vi "Fetch Multiple Records.vi"(0 "device session in":refnum<class "Device Session.lvclass">, 1 "starting record":u64, 2 "number of records":u64=1, 5 "fetch relative to":T1=enum."First Pretrigger Sample", 7 "number of samples":u64=1000, 9 "timeout (ms)":i32=1000, 11 "error in":errorcluster, 12 "fetch offset":i64) -> (4 "device session out":refnum<class "Device Session.lvclass">, 6 "data":dbl[][](array[numeric]), 8 "relativeX (samples)":dbl[](array[numeric]), 14 "requested records info":T2[](array[typedef]), 15 "error out":errorcluster)   [LabVIEW 2021, in "Device Session.lvclass"]
doc: "Fetches data from multiple records in an acquisition. No data is returned if this VI times out. You must run the <B>Initiate</B> VI before running this VI.\n\n<B>Input Parameters</B>\n\n<B>device session in</B> is a reference to the Device Session object, which contains a session to each instrument design library used in this sample project. This parameter is obtained from the 'Open Session' VI.\n\n<B>number of records</B> specifies the number of records to fetch samples from. The default value is 1.\n\n<B>starting record</B> specifies the record to retrieve. Index of the record numbers starts at 0.\n\n<B>fetch relative to</B> specifies the relative location within the acquired record from where the VI begins to fetch data.\n\n'First Sample': the fetch starts at the first sample acquired by the device. If the device wraps data in its memory buffer, the first sample is no longer available. In this case, the VI returns an error if 'fetch offset' specifies a location that is within the overwritten portion of the memory buffer.\n'Reference Trigger Sample': the fetch starts relative to the Reference Trigger.\n'First Pretrigger Sample': the fetch starts relative to the first pretrigger sample acquired. If you do not configure a Reference Trigger, 'First Pretrigger Sample' behaves the same as 'First Sample' because there are no pretrigger samples.\n'Most Recent Sample': the fetch starts relative to the most recently acquired sample. The value of 'fetch offset' must be negative. This VI doesn't support this option. Consider using the 'Fetch Single Record' VI instead.\n'Current Read Position': the fetch starts after the last fetched sample. This VI doesn't support this option. Consider using the 'Fetch Single Record' VI instead.\n\n<B>number of samples</B> specifies the number of samples to fetch. The default value is 1000.\n\n<B>timeout (ms)</B> specifies the time, in milliseconds, allotted for the Fetch Multiple Records VI to complete execution of each record before returning a timeout error. A value of -1 specifies that the VI waits until all data is available. A value of 0 is not supported. The default value is 10,000. You cannot abort a pending fetch using the Abort VI or Close VI.\n\n<B>fetch offset</B> specifies the offset relative to the position, which is specified by the 'fetch relative to' parameter, from which to start fetching data. Offset can be a positive or negative value. The default value is 0.\n\n<B>error in</B> describes error conditions that occur before this node runs. This input provides standard 'error in' functionality.\n\n<B>Output Parameters</B>\n\n<B>device session out</B> passes a reference to the session to the next VI.\n\n<B>data</B> returns the acquired records. Each waveform corresponds to a record. If the fetch contains multiple channels, all waveforms for a record are returned before proceeding to the next record. For example, a two-channel, two-record acquisition returns four waveforms:\narray index 0 = Channel0 Record0\narray index 1 = Channel1 Record0\narray index 2 = Channel0 Record1\narray index 3 = Channel1 Record1\n\n<B>relativeX (samples)</B> returns the relative positions from the trigger to the first sample in the acquired data.\n\n<B>requested records info</B> returns additional information about each record returned by 'data'. There is one element in the 'requested records info' array for each record.\n\n<B>requested records info.number of samples</B> returns the number of samples in the record.\n\n<B>requested records info.starting sample number</B> returns the sample number of the first sample in the returned record data. Sample numbers are zero-based. Sample numbers start at zero for each record and increment by one for each acquired sample.\n\n<B>requested records info.number of channels</B> returns the number of channels in the record data.\n\n<B>requested records info.timestamps</B> returns the timestamp values that were captured for the record.\n\n<B>error out</B> contains error information. This output provides standard 'error out' functionality."
uses:
  Device Session.lvclass
  <instrlib>/_niInstr/Multirecord Acquisition/Interface/v1/Host/Public/Requested Record Info.ctl
  <instrlib>/_niInstr/Multirecord Acquisition/Interface/v1/Host/Public/Fetch Relative To Enum.ctl
  Device Session.lvclass/Device Session.ctl
  <instrlib>/_niInstr/Multirecord Acquisition/Interface/v1/Host/Private/Fetch Multiple Records DBL Wrapper.vi
  <instrlib>/HSAI-RIO/Config/Group A/v1/Host/Main/niHSAI Group A Config v1 Host.lvclass
  <instrlib>/_niInstr/Multirecord Acquisition/Interface/v1/Host/niInstr Multirecord Acquisition v1 Host.lvclass
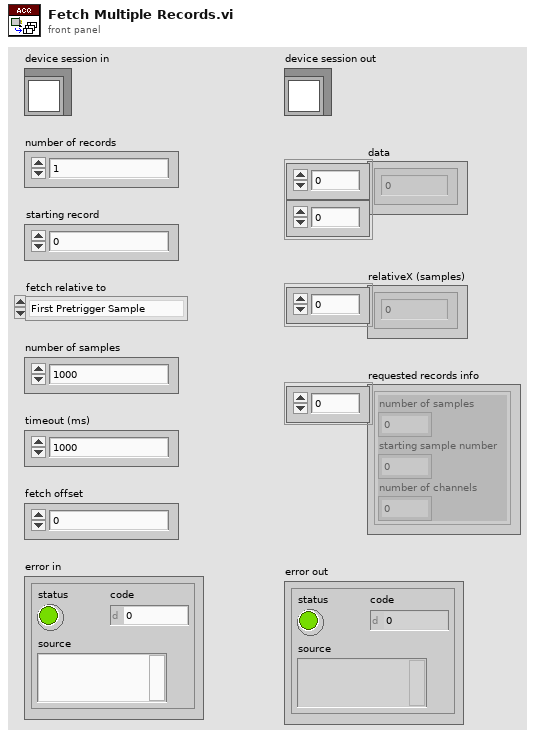
[diagram p1: front panel]
types:
  T1 = typedef "niInstr Multirecord Acquisition v1 Host.lvclass/Fetch Relative To Enum.ctl" = enum16{"First Sample", "Reference Trigger Sample", "First Pretrigger Sample", "Most Recent Sample", "Current Read Position"}
  T2 = typedef "niInstr Multirecord Acquisition v1 Host.lvclass/Requested Record Info.ctl" = cluster{"number of samples":u64, "starting sample number":u64, "number of channels":u64, "timestamps":u64[]}
  T3 = typedef "Device Session.lvclass/Device Session Object.ctl" = cluster{"fpga reference":T4, "reg bus":refnum<class "niInstr FIFO Register Bus v1 Host.lvclass">, "subsystem map":refnum<class "niInstr Subsystem Map v1 Host.lvclass">, "cal data":refnum<class "niHSAI Cal Data v1 Host.lvclass">, "config":refnum<class "niHSAI Group A Config v1 Host.lvclass">, "acquisition":refnum<class "niInstr Multirecord Acquisition v1 Host.lvclass">, "number of selected acq channels":u8, "selected acq channels":bool[], "number of channels":u32, "configured channels":bool[], "acq configuration":cluster{"number of samples":u64, "number of records":u64, "pretrigger samples":u64}, "actual channel configuration":T5[], "sample clock rate (Hz)":dbl, "scaling coefficients":T9[]}
  T4 = typedef "Device Session.lvclass/FPGA Refnum.ctl" = refnum<k20>
  T5 = typedef "niHSAI Types v1 Host.lvlib/Channel Configuration.ctl" = cluster{"channel":u32, "coupling":T6, "impedance":T7, "bandwidth":T8, "vertical range":dbl, "vertical offset":dbl}
  T6 = typedef "niHSAI Types v1 Host.lvlib/Coupling.ctl" = enum8{"Default", "DC", "AC"}
  T7 = typedef "niHSAI Types v1 Host.lvlib/Impedance.ctl" = enum8{"Default", "1 mega ohm", "50 ohm"}
  T8 = typedef "niHSAI Types v1 Host.lvlib/Bandwidth.ctl" = enum8{"Default", "Full Bandwidth", "Anti-alias Filter", "150 MHz"}
  T9 = typedef "niInstr Multirecord Acquisition v1 Host.lvclass/Scaling Coefficient.ctl" = cluster{"gain":dbl, "offset":dbl}
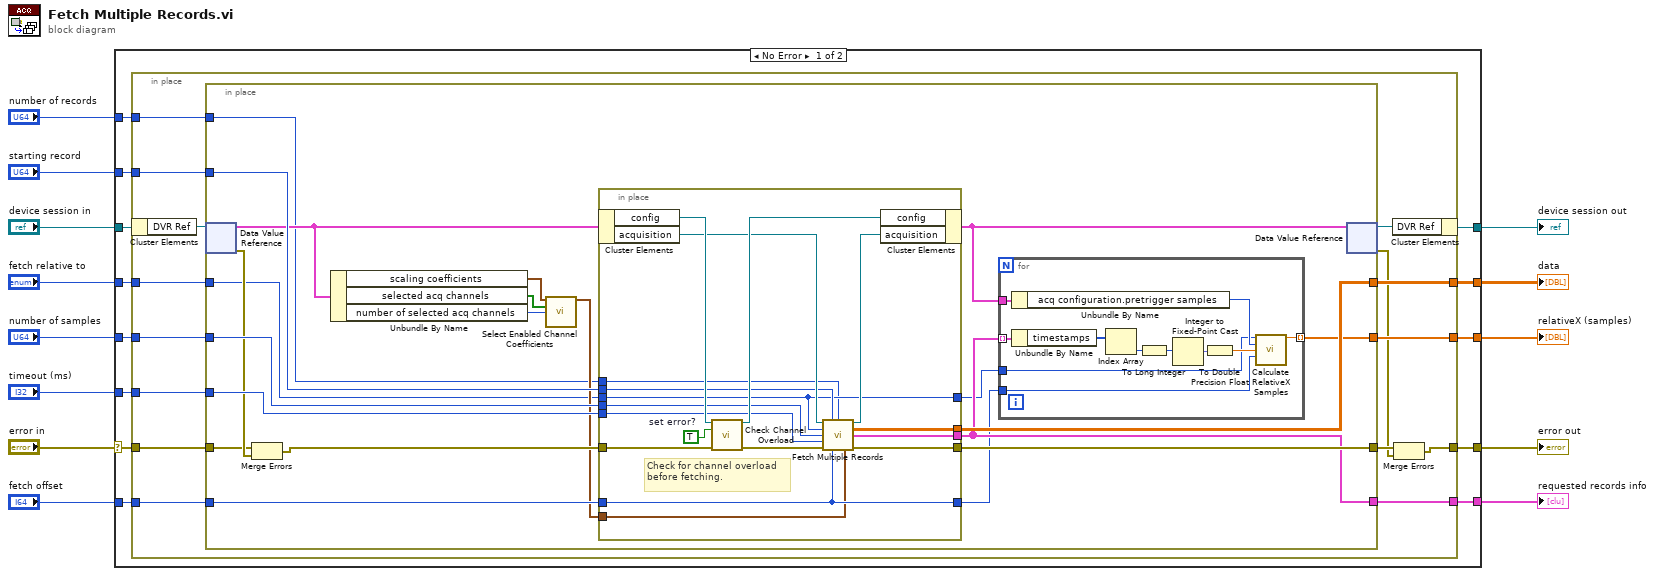
[diagram p0: block diagram]
diagram:
  n1 = case shown="No Error" "error in" {
    selector: "error in" -> [w26 w92]
    tunnel: [w21 w92] -> w1
    tunnel: "device session in" -> [w16 w91]
    tunnel: [w15 w91] -> w5
    tunnel: "number of samples" -> [w25 _]
    tunnel: "timeout (ms)" -> [w24 _]
    tunnel: "fetch offset" -> [w23 _]
    tunnel: "starting record" -> [w22 _]
    tunnel: "fetch relative to" -> [w20 _]
    tunnel: [w19 _] -> w4
    tunnel: [w18 _] -> w2
    tunnel: [w17 _] -> w3
    tunnel: "number of records" -> [w14 _]
    frame No Error {
      n2 = in-place {
        in-place-border: w26 -> [w41]
        in-place-border: w25 -> [w40]
        in-place-border: w24 -> [w39]
        in-place-border: w23 -> [w38]
        in-place-border: w22 -> [w37]
        in-place-border: [w36] -> w21
        in-place-border: w20 -> [w34]
        in-place-border: [w33] -> w19
        in-place-border: [w32] -> w18
        in-place-border: [w31] -> w17
        in-place-border: w14 -> [w27]
        n3 = in-place-cluster #1(w16) -> ("DVR Ref"=w29:refnum<data-value>)
        n4 = in-place {
          in-place-border: w41 -> [w58]
          in-place-border: [w62] -> w35
          in-place-border: w40 -> [w61]
          in-place-border: w39 -> [w60]
          in-place-border: w38 -> [w50]
          in-place-border: w37 -> [w55]
          in-place-border: w34 -> [w47]
          in-place-border: [w54] -> w33
          in-place-border: [w53] -> w32
          in-place-border: [w46] -> w31
          in-place-border: w27 -> [w44]
          n5 = in-place-dvr #2(w29) -> (w48:T3, w59:errorcluster)
          n6 = Merge Errors(w58, w59) -> (w51:errorcluster)
          n7 = Unbundle By Name(w48) -> ("scaling coefficients"=w52:T9[], "selected acq channels"=w57:bool[], "number of selected acq channels"=w56:u8)
          n8 = call "Select Enabled Channel Coefficients.vi"("configured scaling coefficients"=w52, "selected acq channels to store"=w57, "number of selected acq channels to store"=w56) -> ("stored scaling coefficients"=w49:T9[])  [unwired: 12 in]
          n9 = in-place {
            in-place-border: [w90] -> w62
            in-place-border: w61 -> [w79]
            in-place-border: w60 -> [w78]
            in-place-border: w55 -> [w80]
            in-place-border: [w87] -> w54
            in-place-border: [w86] -> w46
            in-place-border: w51 -> [w85]
            in-place-border: w47 -> [w77]
            in-place-border: w50 -> [w76]
            in-place-border: w49 -> [w75]
            in-place-border: [w77] -> w43
            in-place-border: [w76] -> w42
            in-place-border: w44 -> [w74]
            w88 = TRUE  # set error?
            # "Check for channel overload before fetching."
            n10 = in-place-cluster #3(w48) -> ("config"=w84:refnum<class "niHSAI Group A Config v1 Host.lvclass">, "acquisition"=w82:refnum<class "niInstr Multirecord Acquisition v1 Host.lvclass">)
            n11 = call-dynamic "Check Channel Overload.vi"("session in"=w84, "set error? (T)"=w88, "error in"=w85) -> ("session out"=w83:refnum<class "niHSAI Group A Config v1 Host.lvclass">, "error out"=w89:errorcluster)  [unwired: 10 in, 1 out]
            n12 = call-poly <instrlib>:"Fetch Multiple Records.vi"("session in"=w82, "starting record"=w80, "number of records"=w74, "fetch relative to"=w77, "number of samples"=w79, "timeout (ms)"=w78, "error in"=w89, "fetch offset"=w76, "scaling coefficients"=w75) -> ("session out"=w81:refnum<class "niInstr Multirecord Acquisition v1 Host.lvclass">, "data"=w87:dbl[][], "requested records info"=w86:T2[], "error out"=w90:errorcluster)  [unwired: 3 in]
            n13 = in-place-cluster #3("config"=w83, "acquisition"=w81) -> (w45:T3)
          }
          n14 = for {
            tunnel: [w73] -> w53 mode=indexing
            tunnel: w46 -> [w68] mode=indexing
            tunnel: w45 -> [w66]
            tunnel: w43 -> [w64]
            tunnel: w42 -> [w63]
            n15 = Unbundle By Name(w66) -> ("acq configuration.pretrigger samples"=w65:u64)
            n16 = Unbundle By Name(w68) -> ("timestamps"=w70:u64[])
            n17 = Index Array(array=w70) -> (element=w69:u64)  [unwired: 1 in]
            n18 = To Long Integer(number=w69) -> (32bit integer=w71:i32)
            n19 = Integer to Fixed-Point Cast(integer=w71) -> (fixed-point=w72:fxp<+/-,32,5>)  [unwired: 1 in]
            n20 = To Double Precision Float(number=w72) -> (double precision float=w67:dbl)
            n21 = call "Calculate RelativeX Samples.vi"("fetch relative to"=w64, "pretrigger samples"=w65, "timestamps"=w67, "fetch offset"=w63) -> ("relativeX (samples)"=w73:dbl)  [unwired: 11 in]
          }
          n22 = in-place-dvr #2(w45) -> (w28:refnum<data-value>, w30:errorcluster)
        }
        n23 = in-place-cluster #1("DVR Ref"=w28) -> (w15:refnum<class "Device Session.lvclass">)
        n24 = Merge Errors(w35, w30) -> (w36:errorcluster)
      }
    }
    frame Error {
    }
  }
  "error out" <- w1
  "device session out" <- w5
  "requested records info" <- w3
  "data" <- w4
  "relativeX (samples)" <- w2
